vi "點檢_VI_找圓.vi"(8 "error in (no error)":errorcluster, 10 "ROI Descriptor":T2 {"Contours"."Type" items=["No Selection", "Point", "Line", "Rectangle", "Oval", "Polygon", "Free", "Annulus", "Unused2", "Unused3", "Broken Line", "Free Hand Line", "Rotated Rectangle"]}, 11 "Image":T1) -> (0 "error out":errorcluster, 1 "半徑 (Pixels)":dbl, 2 "圓心 (Pixels)":cluster{"X":sgl, "Y":sgl}, 3 "Image Out":T1)   [LabVIEW 2015]
uses:
  <vilib>/vision/Image Controls.llb/IMAQ Image.ctl
  <vilib>/vision/NI_Vision_Development_Module.lvlib
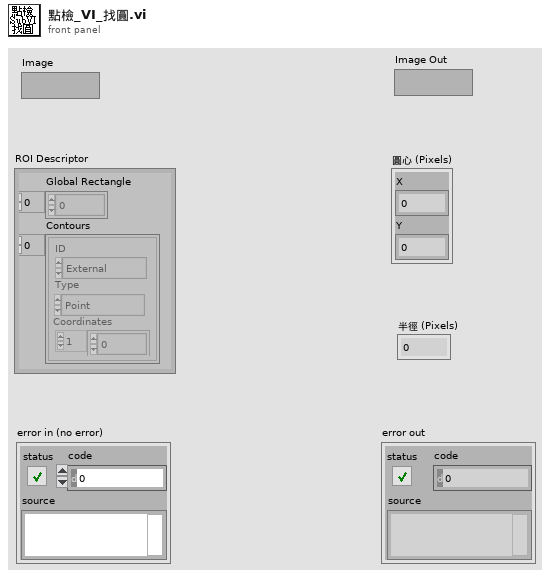
[diagram p1: front panel]
types:
  T1 = typedef "IMAQ Image.ctl" = refnum<image>
  T2 = cluster{"Global Rectangle":i32[], "Contours":cluster{"ID":enum32{"External", "Internal"}, "Type":u32, "Coordinates":i32[]}[]}
  T3 = cluster{"Center (Pixels)":cluster{"X":sgl, "Y":sgl}, "Radius (Pixels)":dbl, "Center (Real-World)":cluster{"X":sgl, "Y":sgl}, "Radius (Real-World)":dbl, "Roundness (Real-World)":dbl, "Average Strength":dbl, "Average SNR (dB)":dbl}
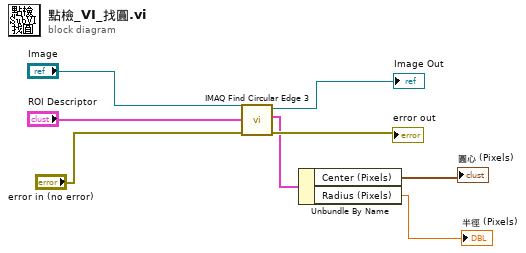
[diagram p0: block diagram]
diagram:
  n1 = call "IMAQ Find Circular Edge 3"("error in (no error)"="error in (no error)", "ROI Descriptor"="ROI Descriptor", "Image"="Image") -> ("error out"=→"error out":errorcluster, "Fitted Circle"=w6:T3, "Image Out"=→"Image Out":T1)  [unwired: 4 in, 2 out]
  n2 = Unbundle By Name(w6) -> ("Center (Pixels)"=→"圓心 (Pixels)":cluster{"X":sgl, "Y":sgl}, "Radius (Pixels)"=→"半徑 (Pixels)":dbl)
